vi "Báscula.vi"() -> ()   [LabVIEW 2018]
panel:
  out "Diferencia":u32
  out "Valor de B":u32
  out "Valor de A":u32
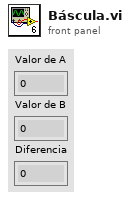
[diagram p1: front panel]
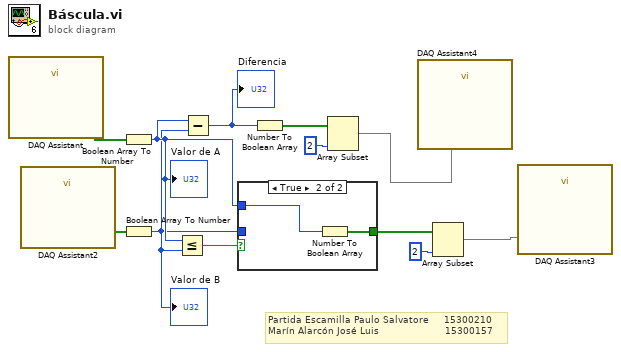
[diagram p0: block diagram]
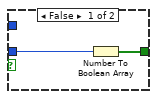
[diagram p2: hidden frame]
diagram:
  # "Partida Escamilla Paulo Salvatore     15300210\nMarín Alarcón José Luis                      15300157"
  n1 = call "DAQ Assistant"() -> ("data"=w12:bool[])  [unwired: 17 in, 2 out]
  n2 = call "DAQ Assistant2"() -> ("data"=w11:bool[])  [unwired: 17 in, 2 out]
  n3 = Boolean Array To Number(Boolean array=w12) -> (number=w9:u32)
  "Valor de A" <- w9
  n4 = Boolean Array To Number(Boolean array=w11) -> (number=w8:u32)
  "Valor de B" <- w8
  n5 = Less Or Equal?(x=w9, y=w8) -> (x <= y?=w10:bool)
  n6 = Subtract(x=w9, y=w8) -> (x-y=w7:u32)
  "Diferencia" <- w7
  n7 = case shown="True" w10 {
    tunnel: w9 -> [_ w16]
    tunnel: [w13 w15] -> w6
    tunnel: w8 -> [w14 _]
    frame False {
      n8 = Number To Boolean Array(number=w14) -> (Boolean array=w13:bool[])
    }
    frame True {
      n9 = Number To Boolean Array(number=w16) -> (Boolean array=w15:bool[])
    }
  }
  n10 = Number To Boolean Array(number=w7) -> (Boolean array=w3:bool[])
  n11 = Array Subset(array=w3, length=2) -> (w1:bool[])  [unwired: 1 in]
  n12 = call "DAQ Assistant4"("data"=w1) -> ()  [unwired: 17 in, 2 out]
  n13 = Array Subset(array=w6, length=2) -> (w4:bool[])  [unwired: 1 in]
  n14 = call "DAQ Assistant3"("data"=w4) -> ()  [unwired: 17 in, 2 out]
